vi "TestHarnessDPL-DetBoardOnly-MPCR-MP045-03.vi"() -> ()   [LabVIEW 2024]
uses:
  <vilib>/Analysis/6fits.llb/Curve Fitting Criteria.ctl
  <vilib>/Analysis/1siggen.llb/Ramp Pattern by Samples.vi
  <vilib>/Analysis/1siggen.llb/Ramp Pattern by Delta.vi
  <vilib>/Analysis/NI_AALBase.lvlib
  <userlib>/_OpenG.lib/time/time.llb/openg_time.lvlib
  <instrlib>/Detector SCPI/Detector SCPI.lvlib
  <instrlib>/Keithley 24XX/Keithley 24XX.lvlib
  <instrlib>/Keithley 648X Series/Keithley 648X Series.lvlib
  <vilib>/Analysis/NI_AALPro.lvlib
panel:
  out "error out":errorcluster
  out "OpVsCurrent":cluster{"Ramp Pattern":dbl[], dbl[]}[](array[cluster])
  in  "Abort 2":bool
  in  "Exit":bool
  in  "Measurement Mode":T1(tab)
  in  "DetectorData":T2(array[cluster])=[{"Name"="SWIR", "DAC Offset"=1800, "DAC StepsPerHGCount"=26.7}, {"Name"="MWIR", "DAC Offset"=666, "DAC StepsPerHGCount"=4.6}] {"DAC Offset" min=1 max=4095 step=1}
  in  "SPI Clock":i64=1000000
  in  "Oversample":i32=1 min=1 max=4096
  in  "Power":bool=TRUE
  in  "Detector VISA":refnum<visa-resource-name>="Detector_EGSE"
  out "Detector Resource":refnum<visa-resource-name>="COM4"
  out "Voltage (V)":dbl[](array[numeric])=[3.264, 0.0, 12.488, 12.77]
  out "Current (mA)":dbl[](array[numeric])=[0.0, 0.0, 21.6, -3.65]
  in  "ThrowAway":i32=100 min=1 max=10000
  out "Detector EGSE ID String":string="Aberystwyth University,Enfys Detector,#01,v0.5.0\r\n"
  in  "Current source":refnum<visa-resource-name>
  out "BoardTemperature":dbl
  in  "Tab Control":enum32{"Counts", "Temperature"}(tab)
  out "Counts":dbl(graph)=160.194
  out "Temperature":dbl(graph)=160.194
  in  "ResetVDACstats":bool
  in  "Gain":u16(ring) items=["High", "Med", "Low"]
  in  "DAC Value":i32=2076 min=0 max=4095 step=1
  in  "Detector":u16(ring) items=["SWIR", "MWIR"]
  out "Peak-to-Peak (counts)":dbl=0.0026870000001508743 format="%^.4g"
  out "rms (counts) 2":dbl=-2.7284841053187847e-12 format="%^.4g"
  out "Mean Value (counts)":dbl
  out "Elapsed(uS)":i32
  out "size":i32
  in  "Pause":bool
  out "XY Graph":cluster{dbl[], "subarray":dbl[]}(graph)
  in  "Detector 3":u16(ring) items=["SWIR", "MWIR"]
  in  "Gain 3":u16(ring) items=["High", "Med", "Low"]
  in  "trig":dbl=8.0 min=0.0 max=50.0
  in  "DetectorDAC":i32=2076 min=0 max=4095 step=1
  in  "Abort":bool
  out "Output vs current":cluster{"Ramp Pattern":dbl[], dbl[]}[](graph)
  in  "ISweep":bool
  in  "NPoints":i32=10 min=10 max=10000 step=1
  in  "MaxCurrent":dbl=1e-11 min=1e-11 max=1e-06
  in  "MinCurrent":dbl=1e-12 min=-10.0 max=10.0
  in  "Detector 4":u16(ring) items=["SWIR", "MWIR"]
  in  "LogSweep":bool
  in  "Gain 4":u16(ring) items=["High", "Med", "Low"]
  out "slope (counts/nA)":dbl
  out "intercept":dbl
  out "residue":dbl
  out "Max Deviation (counts)":dbl
  in  "DAC":i32 min=0 max=4095 step=1
  in  "Modulation Steps":i32=2 min=2 max=1000 step=1
  in  "Modulation Max":dbl min=0.0 max=10.0
  in  "Modulation Min":dbl min=-10.0 max=10.0
  in  "SweepLight":bool
  in  "Detector 7":u16(ring) items=["SWIR", "MWIR"]
  out "Output vs Light":cluster{dbl[], dbl[]}[](graph)
  in  "Gain 2":u16(ring) items=["High", "Med", "Low"]
  in  "SweepVDAC":bool
  in  "ISource":dbl min=-1e-06 max=1e-06
  in  "VDAC Step":i32=1 min=1 max=100
  in  "VDAC Max":i32 min=0 max=4095
  in  "VDAC Min":i32 min=0 max=4000
  in  "Detector 5":u16(ring) items=["SWIR", "MWIR"]
  out "VDAC Sweep":cluster{dbl[], dbl[]}[](graph)
  in  "Abort SweepVDAC":bool
  in  "Step":bool
  in  "Delay 1 (ms)":i32
  in  "Current 2":dbl
  in  "Current 1":dbl
  out "Step Response":cluster{dbl[], "subarray":dbl[]}(graph)
  in  "chan (0)":i32
  out "exit":bool=TRUE
  # "3.3V supply"
  # "Heater"
  # "+12V Supply"
  # "-12V Supply"
  # "Pause button will halt collection and display.\nThis allows graph to be printed etc."
  # "Burst mode is intended to examine behaviour of the ADC\n\nA burst of readings is recorded on the EGSE and then gathered here."
  # "Light source modulated by USB205L working as voltage source connected to MOD input of LD250C\nreference photodiode monitored by 6846 picoammeter"
  # "Set current to Current#1. Waits for Delay 1 to stabilise, then switches to current 2 and reads 1000 readings as fast as possible"
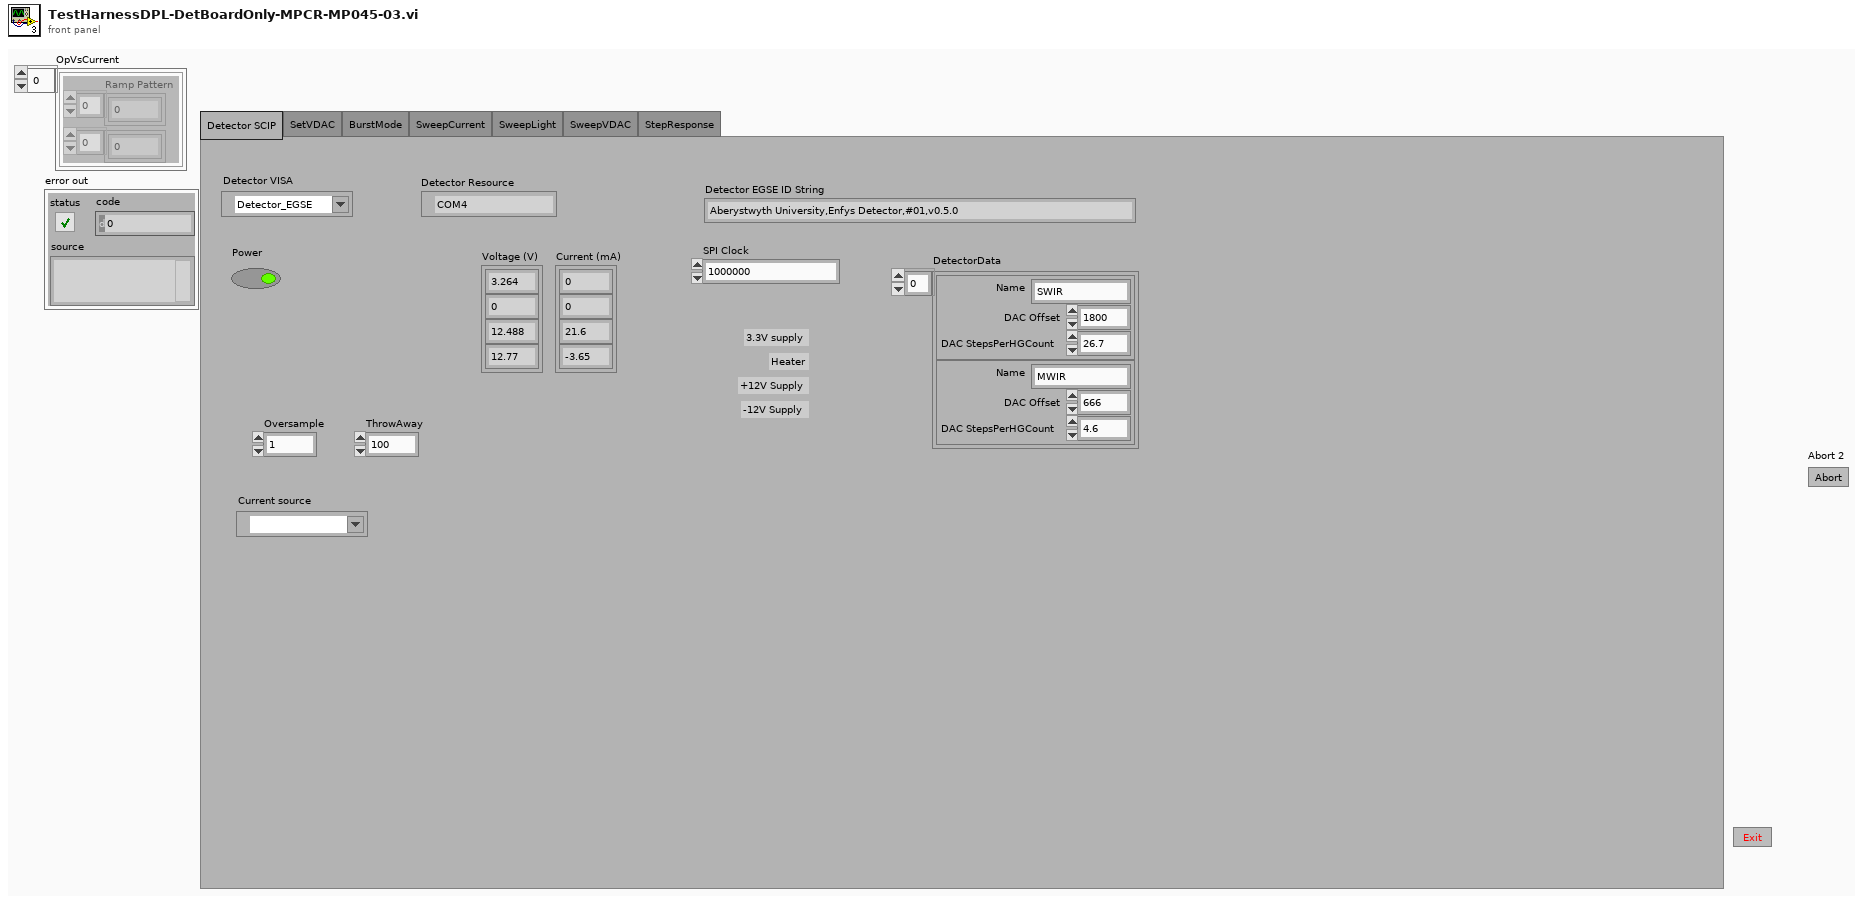
[diagram p1: front panel]
types:
  T1 = enum32{"Detector SCIP", "SetVDAC", "BurstMode", "SweepCurrent", "SweepLight", "SweepVDAC", "StepResponse"}
  T2 = cluster{"Name":string, "DAC Offset":i32, "DAC StepsPerHGCount":dbl}[]
  T3 = cluster{"Baud Rate":u32, "Parity":u16, "Data Bits":u16, "Stop Bits":u16, "Flow Control":u16}
  T4 = cluster{"Name":string, "DAC Offset":i32, "DAC StepsPerHGCount":dbl}
  T5 = typedef "NI_AALPro.lvlib/Curve Fitting Criteria.ctl" = u16
  T6 = typedef "LVPointDoubleTypeDef.ctl" = cluster{"Cursor X":dbl, "Cursor Y":dbl}
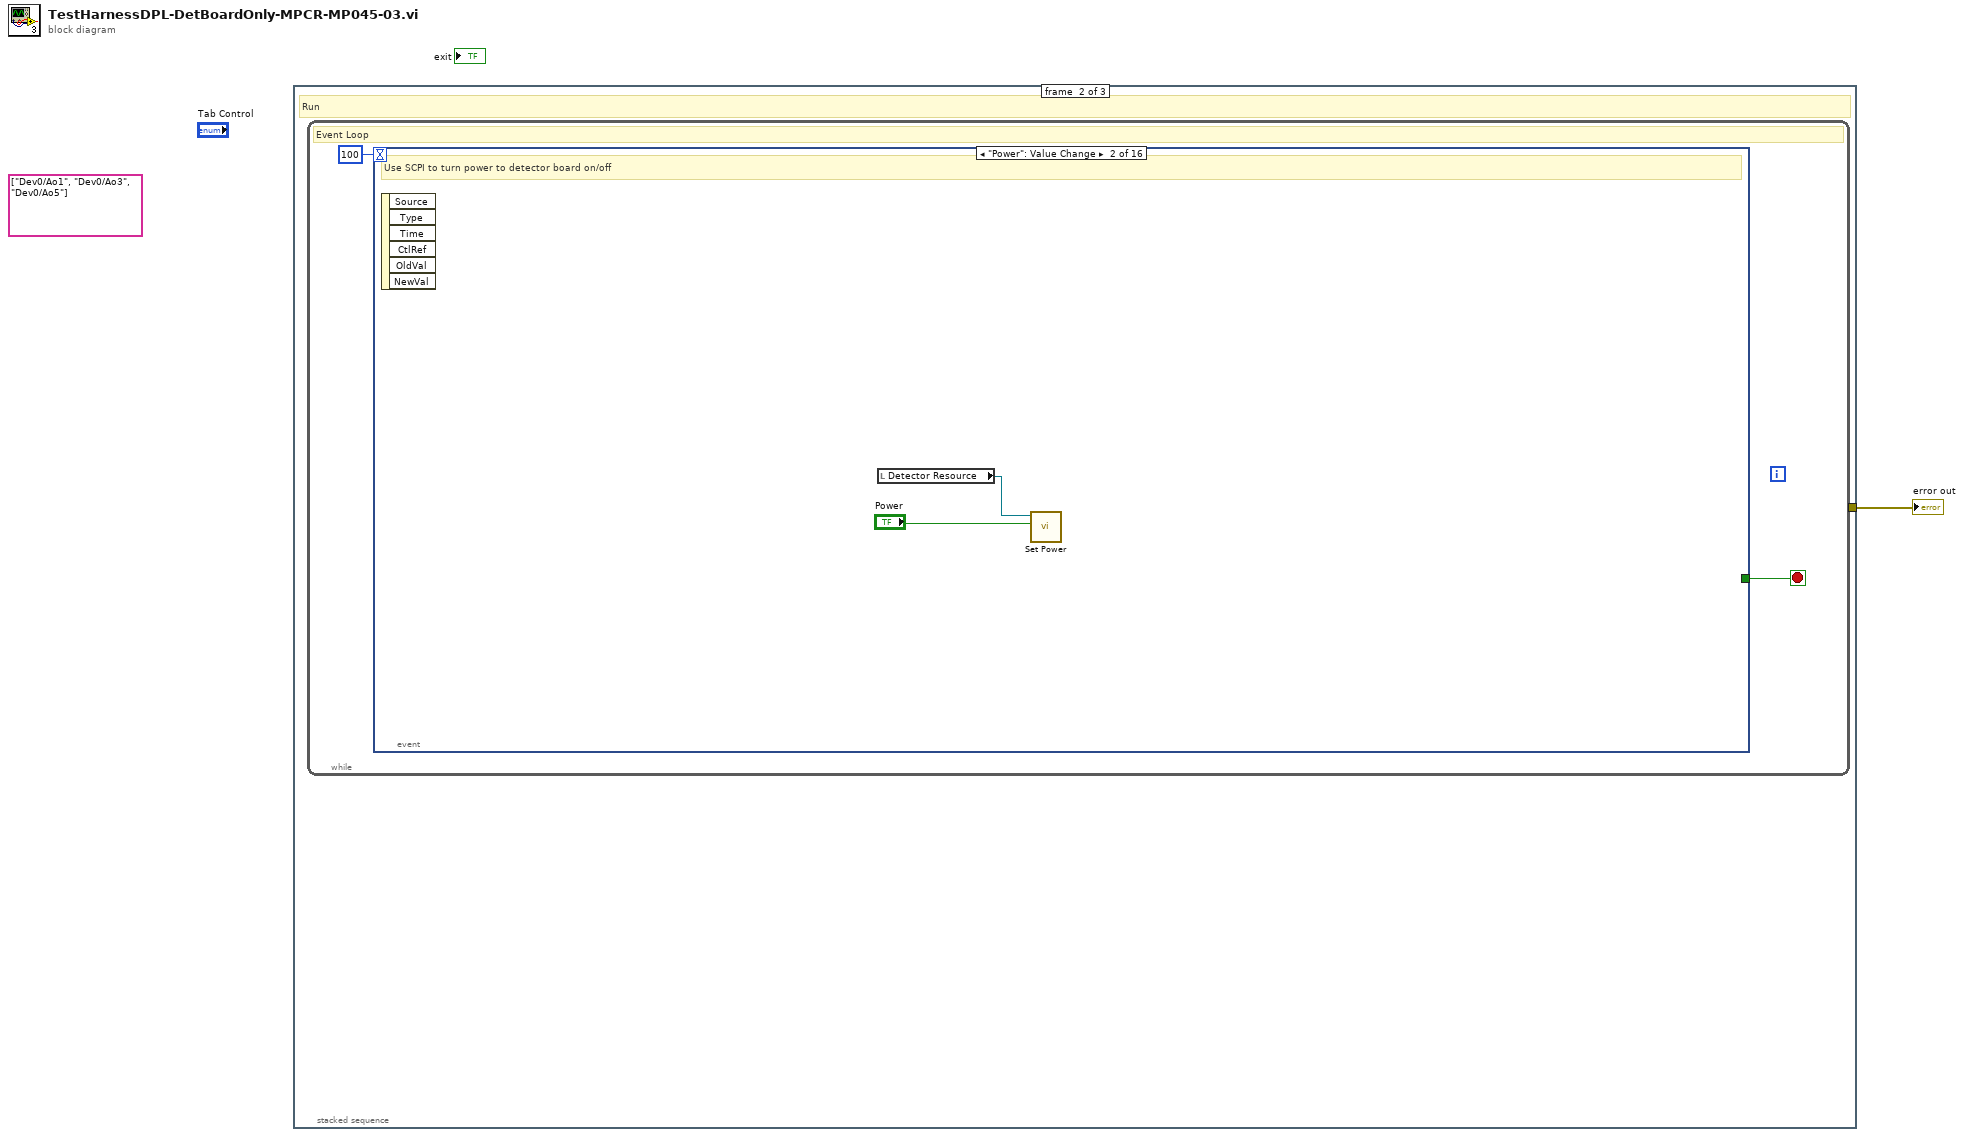
[diagram p0: block diagram]
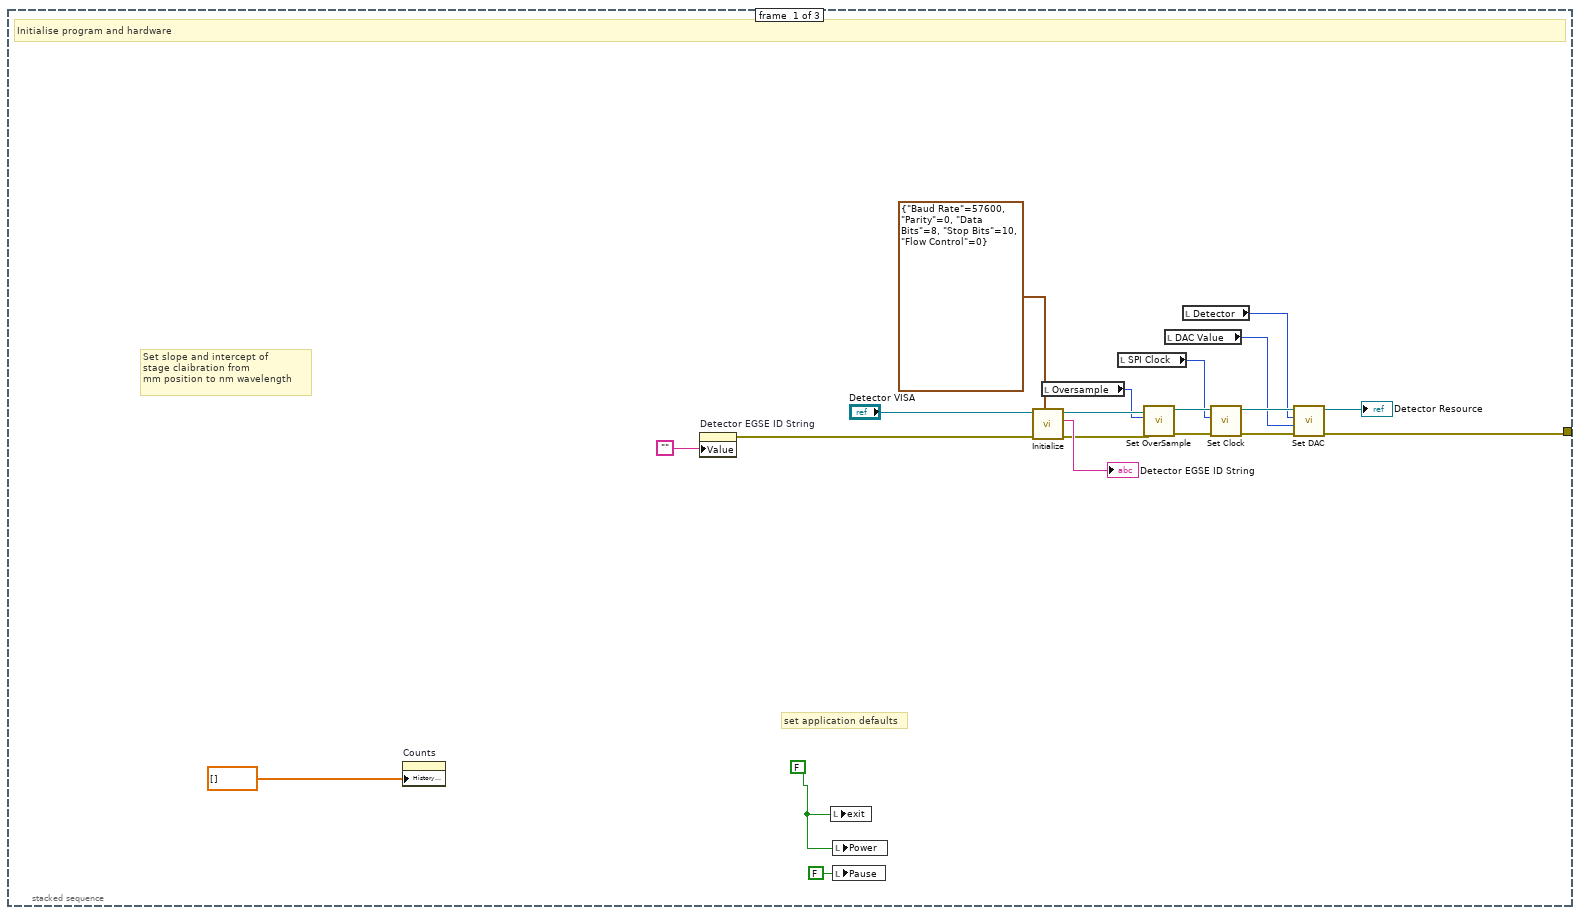
[diagram p2: hidden frame]
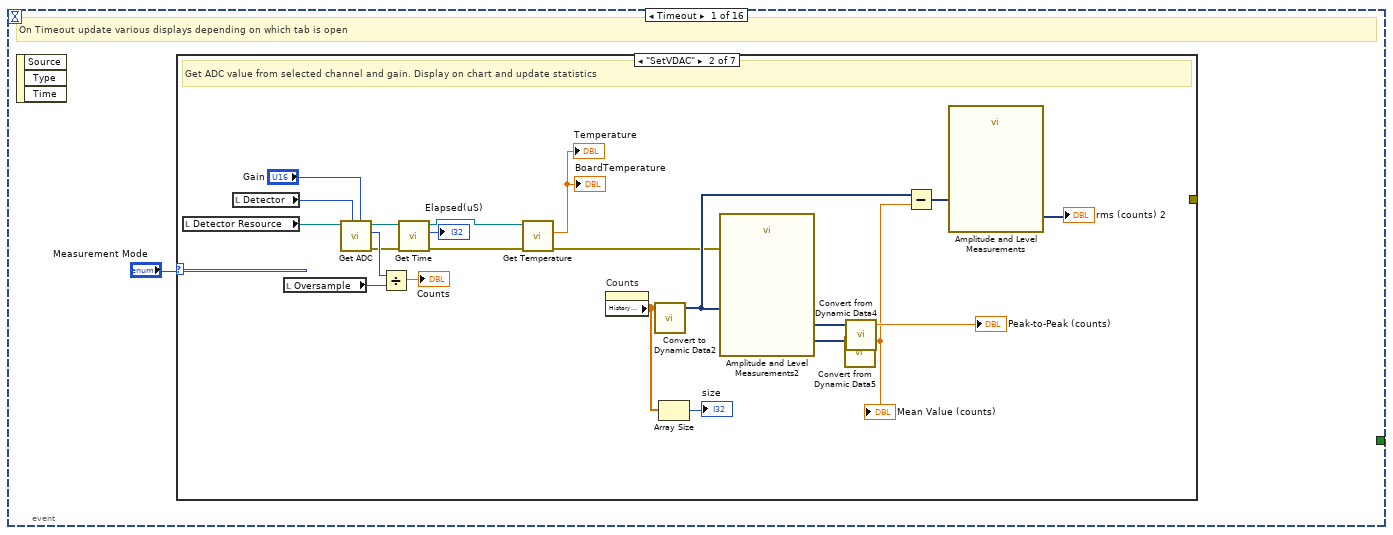
[diagram p3: hidden frame]
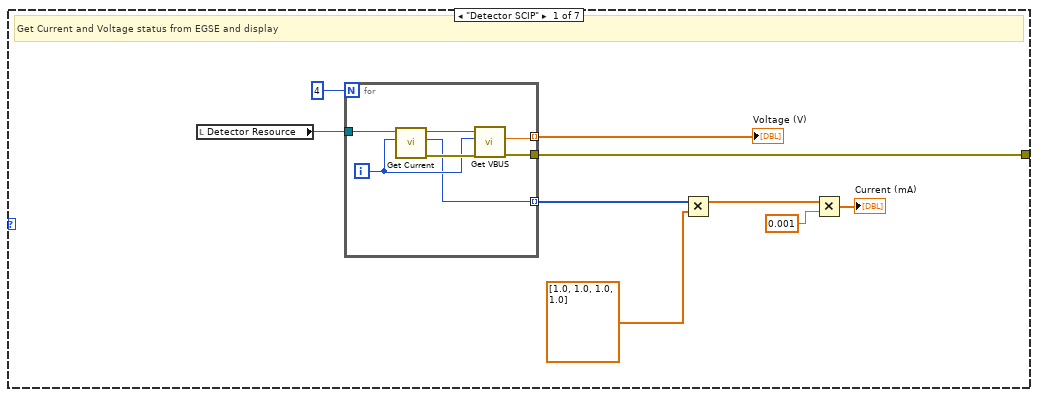
[diagram p4: hidden frame]
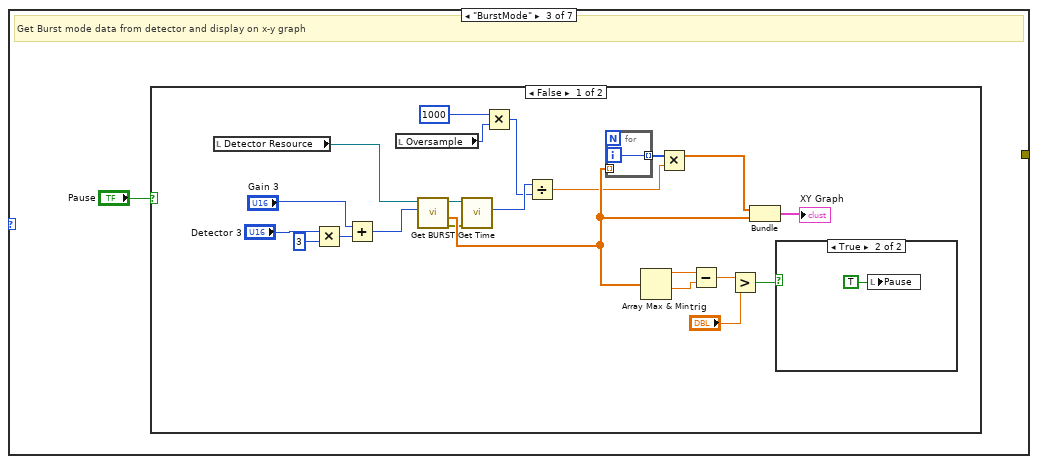
[diagram p5: hidden frame]
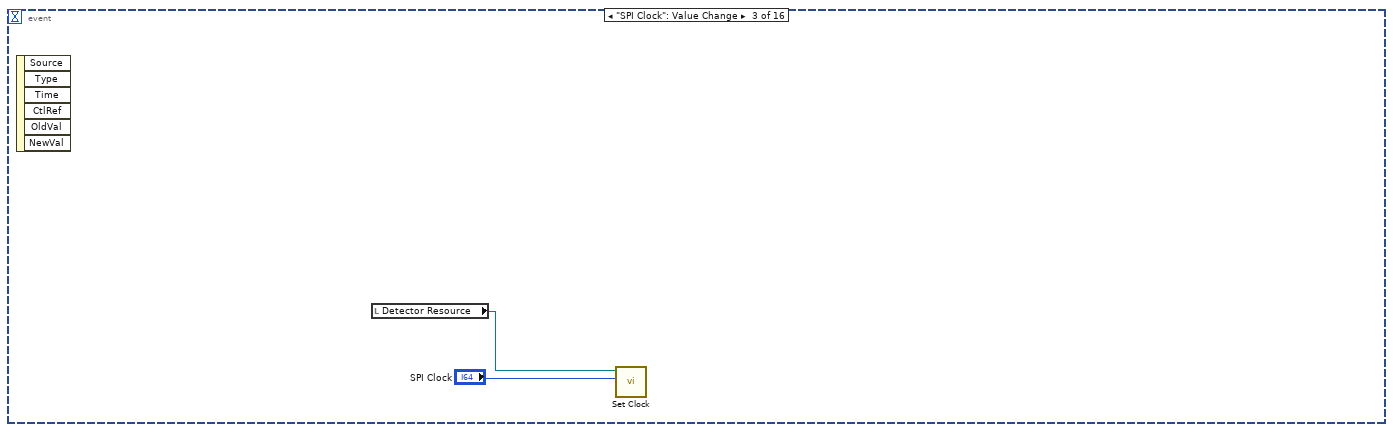
[diagram p12: hidden frame]
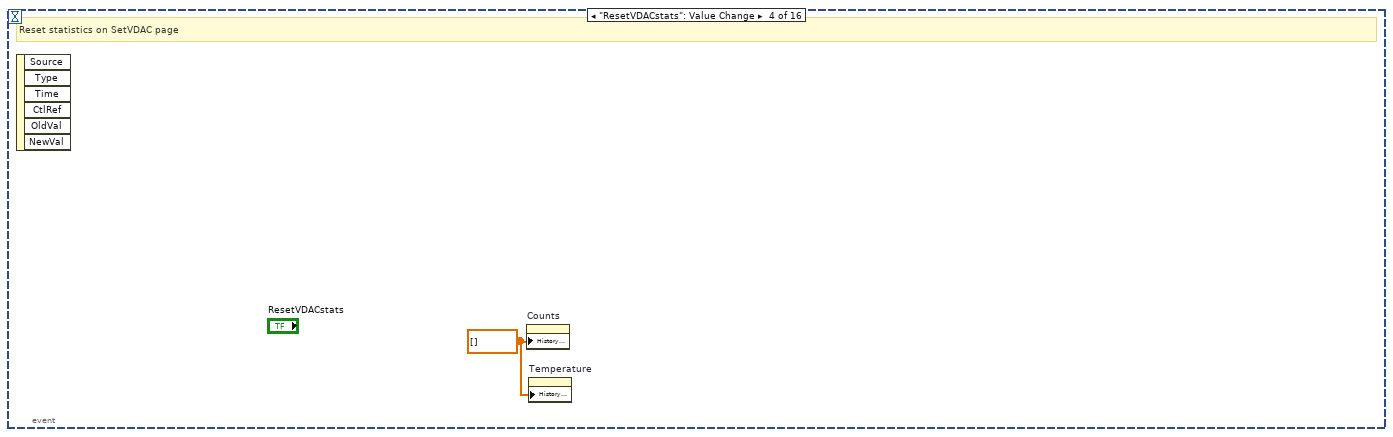
[diagram p13: hidden frame]
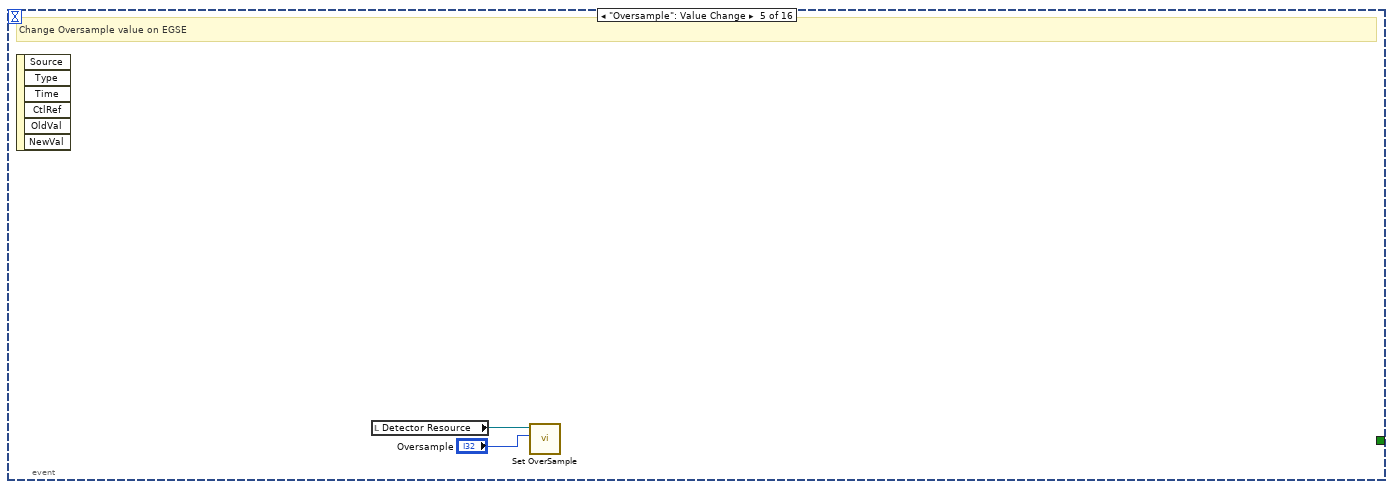
[diagram p14: hidden frame]
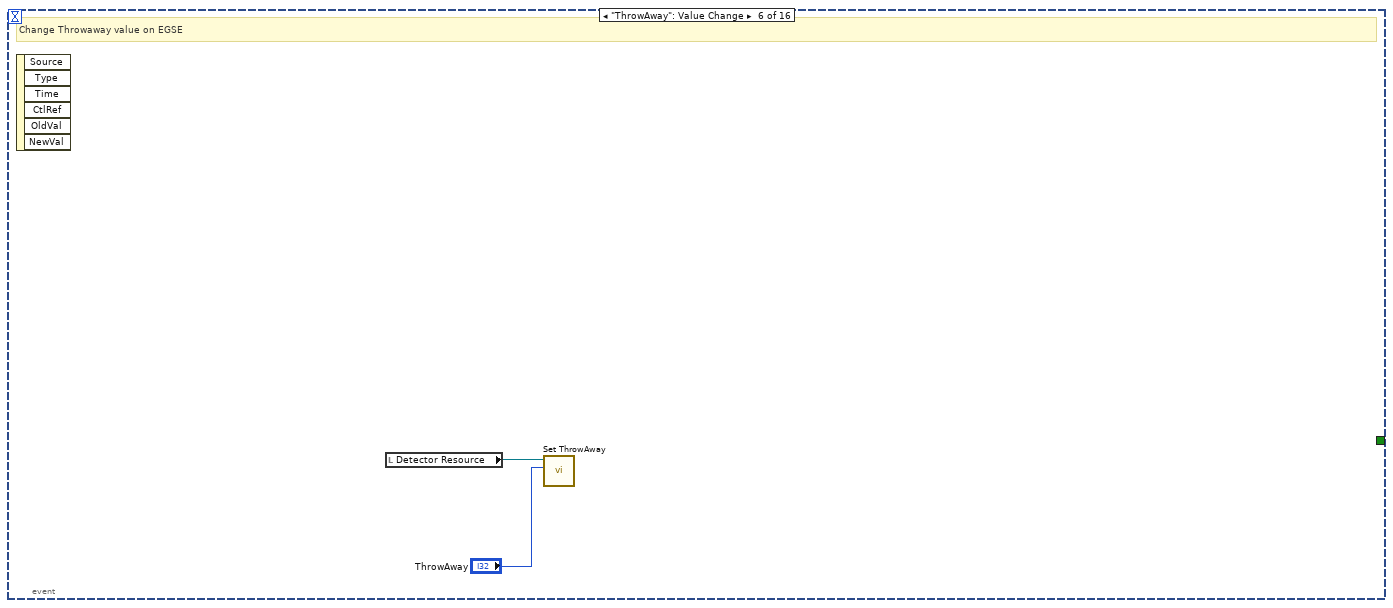
[diagram p15: hidden frame]
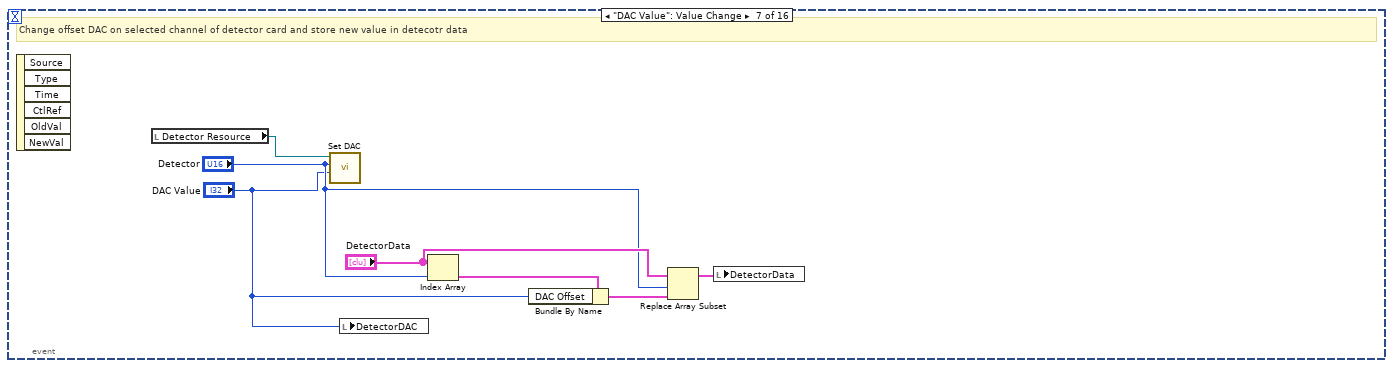
[diagram p16: hidden frame]
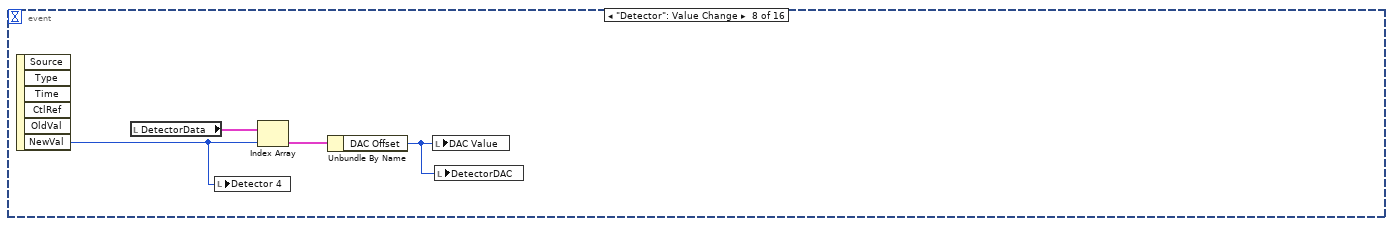
[diagram p17: hidden frame]
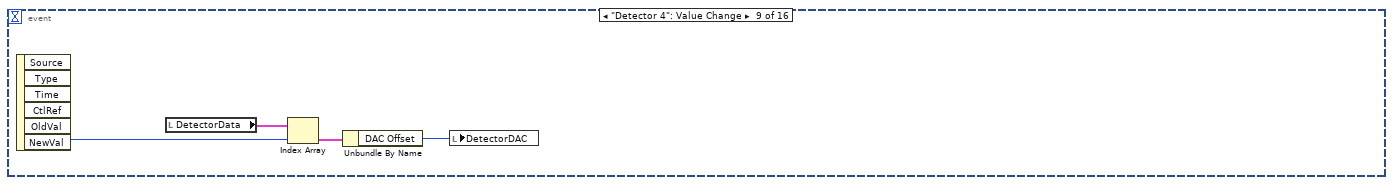
[diagram p18: hidden frame]
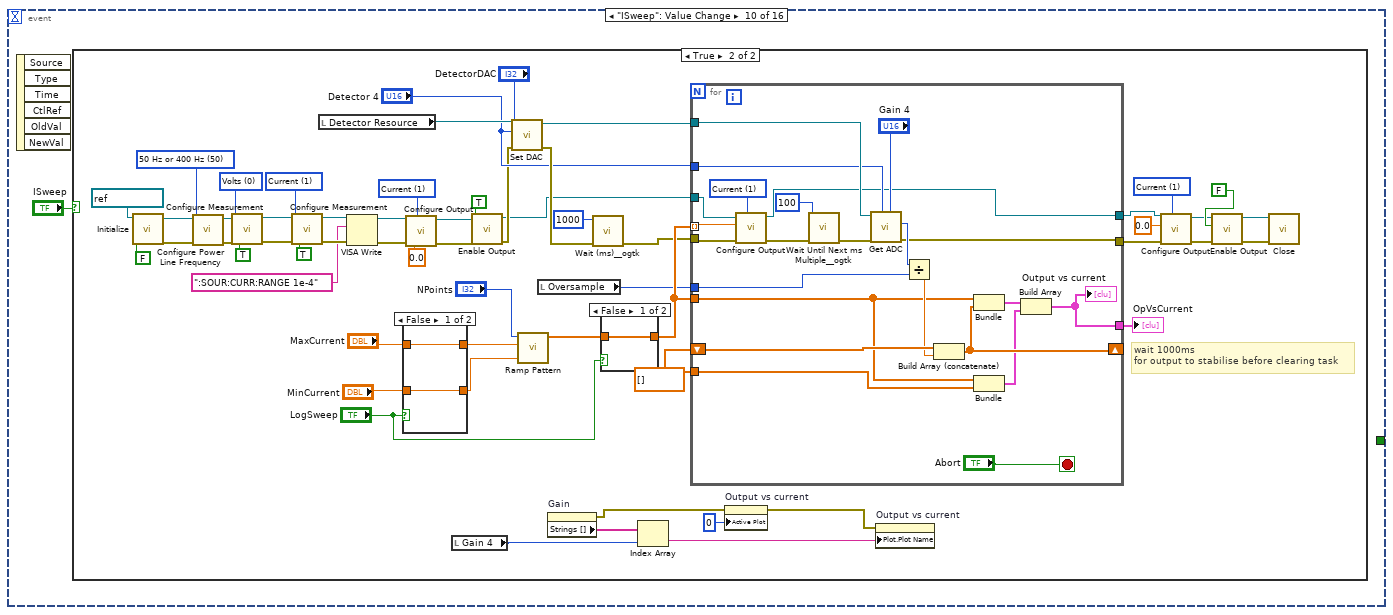
[diagram p19: hidden frame]
diagram:
  (unwired) string[] ["Dev0/Ao1", "Dev0/Ao3", "Dev0/Ao5"]
  n1 = stacked-sequence {
    tunnel: [w2 _ _] -> w1
    frame #0 {
      w20 = FALSE ("connected")
      # "Set slope and intercept of \nstage claibration from\nmm position to nm wavelength"
      # "set application defaults"
      # "Initialise program and hardware"
      n2 = property on="Counts" class="WFChart (strict)"("History Data"=dbl[] []) -> ()  [unwired: 2 in, 2 out]
      n3 = property on="Detector EGSE ID String" class="Str"("Value"="") -> (error out=w18:errorcluster)  [unwired: 2 in, 1 out]
      n4 = local write "exit"(w20) -> ()
      n5 = local write "Power"(w20) -> ()
      n6 = local write "Pause"(FALSE ("Pause")) -> ()
      n7 = call <instrlib>:"Initialize.vi"("Serial Configuration"=T3 {"Baud Rate"=57600, "Parity"=0, "Data Bits"=8, "Stop Bits"=10, "Flow Control"=0}, "error in (no error)"=w18, "VISA resource name"="Detector VISA") -> ("error out"=w14:errorcluster, "ID String"=→"Detector EGSE ID String":string, "VISA resource name out"=w13:refnum<visa-resource-name>)  [unwired: 6 in]
      n8 = local read "Oversample"() -> (w12:i32)
      n9 = local read "SPI Clock"() -> (w7:i64)
      n10 = call <instrlib>:"Set OverSample.vi"("error in (no error)"=w14, "oversample (0)"=w12, "VISA resource name"=w13) -> ("error out"=w11:errorcluster, "VISA resource name out"=w9:refnum<visa-resource-name>)  [unwired: 7 in]
      n11 = local read "DAC Value"() -> (w5:i32)
      n12 = local read "Detector"() -> (w6:u16)
      n13 = call <instrlib>:"Set Clock.vi"("error in (no error)"=w11, "ClockSpeed"=w7, "VISA resource name"=w9) -> ("error out"=w10:errorcluster, "VISA resource name out"=w8:refnum<visa-resource-name>)  [unwired: 7 in]
      n14 = call <instrlib>:"Set DAC.vi"("error in (no error)"=w10, "value (0)"=w5, "chan (0)"=w6, "VISA resource name"=w8) -> ("error out"=w2:errorcluster, "VISA resource name out"=→"Detector Resource":refnum<visa-resource-name>)  [unwired: 6 in]
    }
    frame #1 {
      # "Run"
      n15 = while {
        stop <- w22 stop-if-true
        # "Event Loop"
        n16 = event shown="[1] \"Power\": Value Change" {
          selector: _ -> [_ _ _ _ _ _ _ _ _ _ _ _ _ _ _ _]
          dyn-events: _ -> [_ _ _ _ _ _ _ _ _ _ _ _ _ _ _ _]
          timeout: 100 -> [_ _ _ _ _ _ _ _ _ _ _ _ _ _ _ _]
          tunnel: [_ _ _ _ _ _ _ _ _ _ _ _ _ _ "Exit" _] -> w22
          event Timeout {
            # "On Timeout update various displays depending on which tab is open"
            n17 = event-data() -> ()  [unwired: 1 in, 3 out]
            n18 = case shown="\"SetVDAC\"" "Measurement Mode" {
              tunnel: [w25 _ _ _ _ _ _] -> _
              frame "Detector SCIP" {
                # "Get Current and Voltage status from EGSE and display"
                n19 = local read "Detector Resource"() -> (w33:refnum<visa-resource-name>)
                n20 = for {
                  N: 4 -> [_]
                  tunnel: w33 -> [w40]
                  tunnel: [w36] -> w30 mode=indexing
                  tunnel: [w35] -> w31 mode=indexing
                  tunnel: [w34] -> w25
                  i -> [w37]
                  n21 = call <instrlib>:"Get Current.vi"("chan (1)"=w37, "VISA resource name"=w40) -> ("error out"=w39:errorcluster, "output"=w36:i32, "VISA resource name out"=w38:refnum<visa-resource-name>)  [unwired: 7 in]
                  n22 = call <instrlib>:"Get VBUS.vi"("error in (no error)"=w39, "chan (1)"=w37, "VISA resource name"=w38) -> ("error out"=w34:errorcluster, "output"=w35:dbl)  [unwired: 6 in, 1 out]
                }
                "Voltage (V)" <- w31
                n23 = Multiply(x=w30, y=dbl[] [1.0, 1.0, 1.0, 1.0]) -> (x*y=w27:dbl[])
                n24 = Multiply(x=w27, y=0.001) -> (x*y=→"Current (mA)":dbl[])
              }
              frame "SetVDAC" {
                # "Get ADC value from selected channel and gain. Display on chart and update statistics"
                n25 = local read "Detector Resource"() -> (w62:refnum<visa-resource-name>)
                n26 = local read "Detector"() -> (w57:u16)
                n27 = local read "Oversample"() -> (w59:i32)
                n28 = call <instrlib>:"Get ADC.vi"("Gain"="Gain", "Detector"=w57, "VISA resource name"=w62) -> ("error out"=w55:errorcluster, "output"=w61:i32, "VISA resource name out"=w56:refnum<visa-resource-name>)  [unwired: 6 in]
                n29 = Divide(x=w61, y=w59) -> (x/y=→"Counts":dbl)
                n30 = call <instrlib>:"Get Time.vi"("error in (no error)"=w55, "VISA resource name"=w56) -> ("error out"=w43:errorcluster, "output"=→"Elapsed(uS)":i32, "VISA resource name out"=w41:refnum<visa-resource-name>)  [unwired: 7 in]
                n31 = call <instrlib>:"Get Temperature.vi"("error in (no error)"=w43, "VISA resource name"=w41) -> ("error out"=w42:errorcluster, "output"=→"Temperature" →"BoardTemperature":dbl)  [unwired: 7 in, 1 out]
                n32 = property on="Counts" class="WFChart (strict)"() -> ("History Data"=w46:dbl[])  [unwired: 2 in, 2 out]
                n33 = call "Convert to Dynamic Data2"("Array"=w46) -> ("Dynamic Data Type"=w47:dynamicdata)  [unwired: 3 in]
                n34 = Array Size(array=w46) -> (size(s)=→"size":i32)
                n35 = call "Amplitude and Level Measurements2"("Signals"=w47, "error in (no error)"=w42) -> ("Mean (DC)"=w49:dynamicdata, "Peak to Peak"=w52:dynamicdata)  [unwired: 10 in, 2 out]
                n36 = call "Convert from Dynamic Data5"("Dynamic Data Type"=w49) -> ("Scalar"=w48:dbl)  [unwired: 3 in]
                "Mean Value (counts)" <- w48
                n37 = call "Convert from Dynamic Data4"("Dynamic Data Type"=w52) -> ("Scalar"=→"Peak-to-Peak (counts)":dbl)  [unwired: 3 in]
                n38 = Subtract(x=w47, y=w48) -> (x-y=w50:dynamicdata)
                n39 = call "Amplitude and Level Measurements"("Signals"=w50) -> ("RMS"=→"rms (counts) 2":dynamicdata)  [unwired: 11 in, 3 out]
              }
              frame "BurstMode" {
                # "Get Burst mode data from detector and display on x-y graph"
                n40 = case shown="False" "Pause" {
                  frame False {
                    n41 = local read "Detector Resource"() -> (w85:refnum<visa-resource-name>)
                    n42 = Multiply(x="Detector 3", y=u16 3) -> (x*y=w84:u16)
                    n43 = Add(x="Gain 3", y=w84) -> (x+y=w82:u16)
                    n44 = local read "Oversample"() -> (w69:i32)
                    n45 = call <instrlib>:"Get BURST.vi"("chan (0)"=w82, "VISA resource name"=w85) -> ("error out"=w71:errorcluster, "subarray"=w77:dbl[], "VISA resource name out"=w70:refnum<visa-resource-name>)  [unwired: 6 in, 1 out]
                    n46 = call <instrlib>:"Get Time.vi"("error in (no error)"=w71, "VISA resource name"=w70) -> ("output"=w68:i32)  [unwired: 7 in, 2 out]
                    n47 = Multiply(x=1000, y=w69) -> (x*y=w65:i32)
                    n48 = Divide(x=w68, y=w65) -> (x/y=w66:dbl)
                    n49 = for {
                      tunnel: w77 -> [_] mode=indexing
                      tunnel: [w87] -> w78 mode=indexing
                      i -> [w87]
                    }
                    n50 = Array Max & Min(array=w77) -> (max value=w76:dbl, min value=w75:dbl)  [unwired: 2 out]
                    n51 = Multiply(x=w78, y=w66) -> (x*y=w67:dbl[])
                    n52 = Subtract(x=w76, y=w75) -> (x-y=w74:dbl)
                    n53 = Greater?(x=w74, y="trig") -> (0:w72:bool)
                    n54 = Bundle(w67, "subarray"=w77) -> (→"XY Graph":cluster{dbl[], "subarray":dbl[]})  [unwired: 1 in]
                    n55 = case shown="True" w72 {
                      frame False {
                      }
                      frame True {
                        n56 = local write "Pause"(TRUE ("Pause")) -> ()
                      }
                    }
                  }
                  frame True {
                  }
                }
              }
              frame "SweepCurrent" {
              }
              frame "SweepVDAC" {
              }
              frame "StepResponse" {
              }
              frame "SweepLight" {
              }
            }
          }
          event "Power": Value Change {
            # "Use SCPI to turn power to detector board on/off"
            n57 = event-data() -> ()  [unwired: 1 in, 6 out]
            n58 = local read "Detector Resource"() -> (w89:refnum<visa-resource-name>)
            n59 = call <instrlib>:"Set Power.vi"("Power (0)"="Power", "VISA resource name"=w89) -> ()  [unwired: 8 in, 2 out]
          }
          event "SPI Clock": Value Change {
            n60 = event-data() -> ()  [unwired: 1 in, 6 out]
            n61 = local read "Detector Resource"() -> (w91:refnum<visa-resource-name>)
            n62 = call <instrlib>:"Set Clock.vi"("ClockSpeed"="SPI Clock", "VISA resource name"=w91) -> ()  [unwired: 8 in, 2 out]
          }
          event "ResetVDACstats": Value Change {
            w92 = dbl[] [] ("History Data")
            # "Reset statistics on SetVDAC page"
            n63 = event-data() -> ()  [unwired: 1 in, 6 out]
            n64 = property on="Counts" class="WFChart (strict)"("History Data"=w92) -> ()  [unwired: 2 in, 2 out]
            n65 = property on="Temperature" class="WFChart (strict)"("History Data"=w92) -> ()  [unwired: 2 in, 2 out]
          }
          event "Oversample": Value Change {
            # "Change Oversample value on EGSE"
            n66 = event-data() -> ()  [unwired: 1 in, 6 out]
            n67 = local read "Detector Resource"() -> (w94:refnum<visa-resource-name>)
            n68 = call <instrlib>:"Set OverSample.vi"("oversample (0)"="Oversample", "VISA resource name"=w94) -> ()  [unwired: 8 in, 2 out]
          }
          event "ThrowAway": Value Change {
            # "Change Throwaway value on EGSE"
            n69 = event-data() -> ()  [unwired: 1 in, 6 out]
            n70 = local read "Detector Resource"() -> (w96:refnum<visa-resource-name>)
            n71 = call <instrlib>:"Set ThrowAway.vi"("ThrowAway (0)"="ThrowAway", "VISA resource name"=w96) -> ()  [unwired: 8 in, 2 out]
          }
          event "DAC Value": Value Change {
            # "Change offset DAC on selected channel of detector card and store new value in detecotr data"
            n72 = event-data() -> ()  [unwired: 1 in, 6 out]
            n73 = local read "Detector Resource"() -> (w103:refnum<visa-resource-name>)
            n74 = call <instrlib>:"Set DAC.vi"("value (0)"="DAC Value", "chan (0)"="Detector", "VISA resource name"=w103) -> ()  [unwired: 7 in, 2 out]
            n75 = local write "DetectorDAC"("DAC Value") -> ()
            n76 = Index Array(array="DetectorData", index="Detector") -> (element=w102:T4)
            n77 = Bundle By Name(cluster=w102, "DAC Offset"="DAC Value") -> (w99:T4)
            n78 = Replace Array Subset(array="DetectorData", new element=w99, index="Detector") -> (w98:T2)
            n79 = local write "DetectorData"(w98) -> ()
          }
          event "Detector": Value Change {
            n80 = event-data() -> ("NewVal"=w104:u16)  [unwired: 1 in, 5 out]
            n81 = local read "DetectorData"() -> (w107:T2)
            n82 = local write "Detector 4"(w104) -> ()
            n83 = Index Array(array=w107, index=w104) -> (element=w106:T4)
            n84 = Unbundle By Name(w106) -> ("DAC Offset"=w105:i32)
            n85 = local write "DAC Value"(w105) -> ()
            n86 = local write "DetectorDAC"(w105) -> ()
          }
          event "Detector 4": Value Change {
            n87 = event-data() -> ("NewVal"=w110:u16)  [unwired: 1 in, 5 out]
            n88 = local read "DetectorData"() -> (w111:T2)
            n89 = Index Array(array=w111, index=w110) -> (element=w109:T4)
            n90 = Unbundle By Name(w109) -> ("DAC Offset"=w108:i32)
            n91 = local write "DetectorDAC"(w108) -> ()
          }
          event "ISweep": Value Change {
            n92 = event-data() -> ()  [unwired: 1 in, 6 out]
            n93 = case shown="True" "ISweep" {
              frame False {
              }
              frame True {
                w118 = u16 50 items=["60 Hz"=60, "50 Hz or 400 Hz"=50] ("Power Line Frequency  (60 Hz)")
                w128 = u16 1 items=["Voltage", "Current"] ("Source Mode  (0: Voltage)")
                w137 = u16 1 items=["Volts", "Current", "Resistance"] ("Function (0: Volts)")
                w140 = u16 0 items=["Volts", "Current", "Resistance"] ("Function (0: Volts)")
                w144 = u16 1 items=["Voltage", "Current"] ("Source Mode  (0: Voltage)")
                w155 = dbl[] []
                # "wait 1000ms\nfor output to stabilise before clearing task"
                n94 = call <instrlib>:"Initialize.vi"("ID Query (True)"=FALSE, "VISA resource name"=refnum<visa-resource-name> "B2901BL") -> ("error out"=w119:errorcluster, "VISA resource name out"=w122:refnum<visa-resource-name>)  [unwired: 8 in]
                n95 = call <instrlib>:"Configure Power Line Frequency.vi"("error in (no error)"=w119, "Power Line Frequency  (60 Hz)"=w118, "VISA resource name"=w122) -> ("error out"=w120:errorcluster, "VISA resource name out"=w121:refnum<visa-resource-name>)  [unwired: 7 in]
                n96 = call <instrlib>:"Configure Measurement.vi"("error in (no error)"=w120, "Enable Auto Range (T:Enable)"=TRUE, "Function (0: Volts)"=w140, "VISA resource name"=w121) -> ("error out"=w135:errorcluster, "VISA resource name out"=w136:refnum<visa-resource-name>)  [unwired: 6 in]
                n97 = call <instrlib>:"Configure Measurement.vi"("error in (no error)"=w135, "Enable Auto Range (T:Enable)"=TRUE, "Function (0: Volts)"=w137, "VISA resource name"=w136) -> ("error out"=w117:errorcluster, "VISA resource name out"=w116:refnum<visa-resource-name>)  [unwired: 6 in]
                n98 = local read "Detector Resource"() -> (w162:refnum<visa-resource-name>)
                n99 = VISA Write(VISA resource name=w116, write buffer=":SOUR:CURR:RANGE 1e-4", error in (no error)=w117) -> (VISA resource name out=w115:refnum<visa-resource-name>, error out=w114:errorcluster)  [unwired: 1 out]
                n100 = case shown="False" "LogSweep" {
                  tunnel: "MaxCurrent" -> [w172 w176]
                  tunnel: "MinCurrent" -> [w171 w175]
                  tunnel: [w172 w174] -> w166
                  tunnel: [w171 w173] -> w165
                  frame False {
                  }
                  frame True {
                    n101 = Logarithm Base 10(1:w176) -> (0:w174:dbl)
                    n102 = Logarithm Base 10(1:w175) -> (0:w173:dbl)
                  }
                }
                n103 = call <instrlib>:"Configure Output.vi"("Source Mode  (0: Voltage)"=w144, "error in (no error)"=w114, "Output Level (0)"=0.0, "VISA resource name"=w115) -> ("error out"=w143:errorcluster, "VISA resource name out"=w142:refnum<visa-resource-name>)  [unwired: 6 in]
                n104 = local read "Gain 4"() -> (w147:u16)
                n105 = call <instrlib>:"Enable Output.vi"("error in (no error)"=w143, "Enable Output (T: Enable)"=TRUE ("Auto Output-Off (F: Disable)"), "VISA resource name"=w142) -> ("error out"=w133:errorcluster, "VISA resource name out"=w132:refnum<visa-resource-name>)  [unwired: 7 in]
                n106 = call <instrlib>:"Set DAC.vi"("error in (no error)"=w133, "value (0)"="DetectorDAC", "chan (0)"="Detector 4", "VISA resource name"=w162) -> ("error out"=w157:errorcluster, "VISA resource name out"=w161:refnum<visa-resource-name>)  [unwired: 6 in]
                n107 = call-poly <vilib>:"Ramp Pattern.vi"("start"=w165, "end"=w166, "samples"="NPoints") -> ("Ramp Pattern"=w167:dbl[])  [unwired: 7 in, 1 out]
                n108 = local read "Oversample"() -> (w163:i32)
                n109 = property on="Gain" class="Ring (strict)"() -> (error out=w148:errorcluster, "Strings []"=w153:string[])  [unwired: 2 in, 1 out]
                n110 = call <userlib>:"Wait (ms)__ogtk.vi"("error in (no error)"=w157, "milliseconds to wait"=u32 1000) -> ("error out"=w158:errorcluster)  [unwired: 8 in, 1 out]
                n111 = case shown="False" "LogSweep" {
                  tunnel: w167 -> [w177 w179]
                  tunnel: [w177 w178] -> w164
                  frame False {
                  }
                  frame True {
                    n112 = Power Of 10(x=w179) -> (10^x=w178:dbl[])
                  }
                }
                n113 = Index Array(array=w153, index=w147) -> (element=w149:string)
                n114 = for {
                  tunnel: w158 -> [w193]
                  tunnel: w164 -> [w182] mode=indexing
                  tunnel: [w191] -> w123
                  shift-right: [w199] -> _
                  shift-left: w155 -> [w201]
                  tunnel: w164 -> [w186]
                  tunnel: w161 -> [w198]
                  tunnel: w163 -> [w195]
                  tunnel: "Detector 4" -> [w194]
                  tunnel: [w192] -> w124
                  tunnel: [w184] -> w154
                  tunnel: w155 -> [w185]
                  tunnel: w132 -> [w180]
                  stop <- "Abort" stop-if-true
                  w181 = u16 1 items=["Voltage", "Current"] ("Source Mode  (0: Voltage)")
                  n115 = call <instrlib>:"Configure Output.vi"("Source Mode  (0: Voltage)"=w181, "error in (no error)"=w193, "Output Level (0)"=w182, "VISA resource name"=w180) -> ("error out"=w190:errorcluster, "VISA resource name out"=w192:refnum<visa-resource-name>)  [unwired: 6 in]
                  n116 = call <userlib>:"Wait Until Next ms Multiple__ogtk.vi"("error in (no error)"=w190, "milliseconds to wait"=u32 100) -> ("error out"=w189:errorcluster)  [unwired: 8 in, 1 out]
                  n117 = call <instrlib>:"Get ADC.vi"("Gain"="Gain 4", "Detector"=w194, "error in (no error)"=w189, "VISA resource name"=w198) -> ("error out"=w191:errorcluster, "output"=w200:i32)  [unwired: 5 in, 1 out]
                  n118 = Divide(x=w200, y=w195) -> (x/y=w196:dbl)
                  n119 = Build Array (concatenate)(w201, w196) -> (w199:dbl[])
                  n120 = Bundle("Ramp Pattern"=w186, w199) -> (w187:cluster{"Ramp Pattern":dbl[], dbl[]})  [unwired: 1 in]
                  n121 = Bundle("Ramp Pattern"=w186, w185) -> (w183:cluster{"Ramp Pattern":dbl[], dbl[]})  [unwired: 1 in]
                  n122 = Build Array(w187, w183) -> (w184:cluster{"Ramp Pattern":dbl[], dbl[]}[])
                  "Output vs current" <- w184
                }
                "OpVsCurrent" <- w154
                n123 = property on="Output vs current" class="XYGraph (strict)"(error in=w148, "Active Plot"=u32 0) -> (error out=w150:errorcluster)  [unwired: 1 in, 1 out]
                n124 = property on="Output vs current" class="XYGraph (strict)"(error in=w150, "Plot.Plot Name"=w149) -> ()  [unwired: 1 in, 2 out]
                n125 = call <instrlib>:"Configure Output.vi"("Source Mode  (0: Voltage)"=w128, "error in (no error)"=w123, "Output Level (0)"=0.0, "VISA resource name"=w124) -> ("error out"=w126:errorcluster, "VISA resource name out"=w125:refnum<visa-resource-name>)  [unwired: 6 in]
                n126 = call <instrlib>:"Enable Output.vi"("error in (no error)"=w126, "Enable Output (T: Enable)"=FALSE ("Auto Output-Off (F: Disable)"), "VISA resource name"=w125) -> ("error out"=w130:errorcluster, "VISA resource name out"=w131:refnum<visa-resource-name>)  [unwired: 7 in]
                n127 = call <instrlib>:"Close.vi"("error in (no error)"=w130, "VISA resource name"=w131) -> ()  [unwired: 9 in, 1 out]
              }
            }
          }
          event "Output vs current": Cursor Release {
            w221 = T5 0 items=["Least Square", "Least Absolute Residual", "Bisquare"] ("method")
            n128 = event-data() -> ()  [unwired: 1 in, 9 out]
            n129 = property on="Output vs current" class="XYGraph (strict)"("Active Cursor"=u32 0) -> (error out=w233:errorcluster)  [unwired: 2 in, 1 out]
            n130 = property on="Output vs current" class="XYGraph (strict)"(error in=w233) -> (error out=w230:errorcluster, "Cursor.Cursor Position"=w228:T6)  [unwired: 1 in, 1 out]
            n131 = Unbundle By Name(w228) -> ("Cursor X"=w216:dbl)
            n132 = local read "OpVsCurrent"() -> (w229:cluster{"Ramp Pattern":dbl[], dbl[]}[])
            n133 = property on="Output vs current" class="XYGraph (strict)"(error in=w230, "Active Cursor"=u32 1) -> (error out=w232:errorcluster)  [unwired: 1 in, 1 out]
            n134 = Index Array(array=w229) -> (element=w213:cluster{"Ramp Pattern":dbl[], dbl[]})  [unwired: 1 in]
            n135 = property on="Output vs current" class="XYGraph (strict)"(error in=w232) -> ("Cursor.Cursor Position"=w227:T6)  [unwired: 1 in, 2 out]
            n136 = Unbundle(w213) -> ("Ramp Pattern"=w226:dbl[], w224:dbl[])
            n137 = Unbundle By Name(w227) -> ("Cursor X"=w217:dbl)
            n138 = Max & Min(x=w217, y=w216) -> (max(x,y)=w214:dbl, min(x,y)=w215:dbl)
            n139 = Search 1D Array(1D array=w226, element=w215) -> (index of element=w223:i32)  [unwired: 1 in]
            n140 = local read "Output vs current"() -> (w211:cluster{"Ramp Pattern":dbl[], dbl[]}[])
            n141 = Search 1D Array(1D array=w226, element=w214) -> (index of element=w225:i32)  [unwired: 1 in]
            n142 = Subtract(x=w225, y=w223) -> (x-y=w222:i32)
            n143 = Array Subset(array=w224, index=w223, length=w222) -> (w206:dbl[])
            n144 = Array Subset(array=w226, index=w223, length=w222) -> (w212:dbl[])
            n145 = call <vilib>:"Linear Fit.vi"("Y"=w206, "X"=w212, "method"=w221) -> ("Best Linear Fit"=w207:dbl[], "slope"=→"slope (counts/nA)":dbl, "intercept"=→"intercept":dbl, "residue"=→"residue":dbl)  [unwired: 8 in, 1 out]
            n146 = Bundle(w212, "Best Linear Fit"=w207) -> (w209:cluster{dbl[], "Best Linear Fit":dbl[]})  [unwired: 1 in]
            n147 = Replace Array Subset(array=w211, new element=w209, index=1) -> (w208:cluster{"Ramp Pattern":dbl[], dbl[]}[])
            n148 = Subtract(x=w206, y=w207) -> (x-y=w205:dbl[])
            n149 = local write "Output vs current"(w208) -> ()
            n150 = Absolute Value(x=w205) -> (abs(x)=w204:dbl[])
            n151 = Array Max & Min(array=w204) -> (max value=→"Max Deviation (counts)":dbl)  [unwired: 3 out]
          }
          event "SweepLight": Value Change {
            n152 = event-data() -> ()  [unwired: 1 in, 6 out]
            n153 = case shown="True" "SweepLight" {
              frame False {
              }
              frame True {
                w252 = dbl[] []
                n154 = local read "Detector Resource"() -> (w261:refnum<visa-resource-name>)
                n155 = call "Keithley 648X Series SetupAcquisition.vi"("VISA resource name"=refnum<visa-resource-name> "Picoammeter") -> ("VISA resource name out"=w253:refnum<visa-resource-name>)  [unwired: 8 in, 1 out]
                n156 = local read "Oversample"() -> (w262:i32)
                n157 = call-poly <vilib>:"Ramp Pattern.vi"("start"="Modulation Min", "end"="Modulation Max", "samples"="Modulation Steps") -> ("Ramp Pattern"=w257:dbl[])  [unwired: 7 in, 1 out]
                n158 = call <instrlib>:"Set DAC.vi"("value (0)"="DAC", "chan (0)"="Detector 7", "VISA resource name"=w261) -> ("error out"=w251:errorcluster, "VISA resource name out"=w260:refnum<visa-resource-name>)  [unwired: 7 in]
                n159 = call <instrlib>:"ULx Create Channel (AO-Voltage-Basic).vi"("maximum value"=5.0, "minimum value"=0.0, "physical channels"=refnum<k21> "Dev0/Ao0", "error in"=w251) -> ("task out"=w246:refnum<k24>, "error out"=w245:errorcluster)  [unwired: 10 in]
                n160 = call <instrlib>:"ULx Write (Analog 1D DBL 1Chan 1Samp).vi"("task in"=w246, "data"="Modulation Min", "error in"=w245) -> ("task out"=w247:refnum<k24>, "error out"=w242:errorcluster)  [unwired: 10 in, 1 out]
                n161 = call <userlib>:"Wait (ms)__ogtk.vi"("error in (no error)"=w242, "milliseconds to wait"=u32 1000) -> ("error out"=w243:errorcluster)  [unwired: 8 in, 1 out]
                n162 = for {
                  tunnel: w243 -> [w291]
                  tunnel: [w290] -> w237
                  tunnel: [w272] -> w239
                  shift-right: [w285] -> _
                  shift-left: w252 -> [w287]
                  tunnel: w260 -> [w284]
                  shift-right: [w280] -> _
                  shift-left: w252 -> [w282]
                  shift-right: [w279] -> _
                  shift-left: w252 -> [w281]
                  tunnel: w262 -> [w274]
                  tunnel: "Detector 7" -> [w273]
                  tunnel: w257 -> [w265] mode=indexing
                  tunnel: w253 -> [w271]
                  shift-right: [w267] -> _
                  shift-left: w252 -> [w268]
                  tunnel: w247 -> [w266]
                  stop <- "Abort 2" stop-if-true
                  n163 = call <instrlib>:"ULx Write (Analog 1D DBL 1Chan 1Samp).vi"("task in"=w266, "data"=w265, "error in"=w291) -> ("task out"=w290:refnum<k24>, "error out"=w289:errorcluster)  [unwired: 10 in, 1 out]
                  n164 = call <instrlib>:"Get ADC.vi"("Gain"="Gain 2", "Detector"=w273, "error in (no error)"=w289, "VISA resource name"=w284) -> ("error out"=w283:errorcluster, "output"=w286:i32)  [unwired: 5 in, 1 out]
                  n165 = Divide(x=w286, y=w274) -> (x/y=w263:dbl)
                  n166 = Divide(x=w273, y=w274) -> ()  [unwired: 1 out]
                  n167 = Build Array (concatenate)(w282, w263) -> (w280:dbl[])
                  n168 = Build Array (concatenate)(w287, w263) -> (w285:dbl[])
                  n169 = Build Array (concatenate)(w281, w263) -> (w279:dbl[])
                  n170 = call <instrlib>:"Measure Current.vi"("VISA resource name"=w271, "error in (no error)"=w283) -> ("Measurement"=w269:dbl, "error out"=w272:errorcluster)  [unwired: 11 in, 1 out]
                  n171 = Negate(x=w269) -> (-x=w264:dbl)
                  n172 = Build Array (concatenate)(w268, w264) -> (w267:dbl[])
                  n173 = Bundle(w267, w285) -> (w278:cluster{dbl[], dbl[]})  [unwired: 1 in]
                  n174 = Bundle(w267, w280) -> (w277:cluster{dbl[], dbl[]})  [unwired: 1 in]
                  n175 = Bundle(w267, w279) -> (w276:cluster{dbl[], dbl[]})  [unwired: 1 in]
                  n176 = Build Array(w278, w277, w276) -> (→"Output vs Light":cluster{dbl[], dbl[]}[])
                }
                n177 = call <instrlib>:"ULx Write (Analog 1D DBL 1Chan 1Samp).vi"("task in"=w237, "data"=0.0, "error in"=w239) -> ("task out"=w238:refnum<k24>, "error out"=w240:errorcluster)  [unwired: 10 in, 1 out]
                n178 = call <instrlib>:"ULx Clear Task.vi"("task in"=w238, "error in"=w240) -> ()  [unwired: 13 in, 1 out]
              }
            }
          }
          event "SweepVDAC": Value Change {
            n179 = event-data() -> ()  [unwired: 1 in, 6 out]
            n180 = case shown="True" "SweepVDAC" {
              frame False {
              }
              frame True {
                w305 = u16 1 items=["Voltage", "Current"] ("Source Mode  (0: Voltage)")
                w307 = dbl[] []
                w320 = u16 1 items=["Voltage", "Current"] ("Source Mode  (0: Voltage)")
                w324 = u16 1 items=["Volts", "Current", "Resistance"] ("Function (0: Volts)")
                w326 = u16 0 items=["Volts", "Current", "Resistance"] ("Function (0: Volts)")
                n181 = call <instrlib>:"Initialize.vi"("ID Query (True)"=FALSE, "VISA resource name"="Current source") -> ("error out"=w312:errorcluster, "VISA resource name out"=w313:refnum<visa-resource-name>)  [unwired: 8 in]
                n182 = call <instrlib>:"Configure Measurement.vi"("error in (no error)"=w312, "Enable Auto Range (T:Enable)"=TRUE, "Function (0: Volts)"=w326, "VISA resource name"=w313) -> ("error out"=w327:errorcluster, "VISA resource name out"=w328:refnum<visa-resource-name>)  [unwired: 6 in]
                n183 = call <instrlib>:"Configure Measurement.vi"("Manual Range (1.0)"=1e-07, "error in (no error)"=w327, "Enable Auto Range (T:Enable)"=FALSE, "Function (0: Volts)"=w324, "VISA resource name"=w328) -> ("error out"=w322:errorcluster, "VISA resource name out"=w321:refnum<visa-resource-name>)  [unwired: 5 in]
                n184 = call-poly <vilib>:"Ramp Pattern.vi"("start"="VDAC Min", "end"="VDAC Max", "delta"="VDAC Step") -> ("Ramp Pattern"=w309:dbl[])  [unwired: 6 in, 2 out]
                n185 = local read "Oversample"() -> (w306:i32)
                n186 = local read "Detector Resource"() -> (w308:refnum<visa-resource-name>)
                n187 = call <instrlib>:"Configure Output.vi"("Source Mode  (0: Voltage)"=w320, "error in (no error)"=w322, "Output Level (0)"="ISource", "VISA resource name"=w321) -> ("error out"=w319:errorcluster, "VISA resource name out"=w318:refnum<visa-resource-name>)  [unwired: 6 in]
                n188 = call <instrlib>:"Enable Output.vi"("error in (no error)"=w319, "Enable Output (T: Enable)"=TRUE, "VISA resource name"=w318) -> ("error out"=w315:errorcluster, "VISA resource name out"=w316:refnum<visa-resource-name>)  [unwired: 7 in]
                n189 = for {
                  tunnel: w316 -> [w332]
                  tunnel: w315 -> [w363]
                  tunnel: w309 -> [w362] mode=indexing
                  tunnel: [w332] -> w304
                  tunnel: [w354] -> w302
                  shift-right: [w357] -> _
                  shift-left: w307 -> [w359]
                  tunnel: w309 -> [w345]
                  tunnel: w308 -> [w331]
                  shift-right: [w347] -> _
                  shift-left: w307 -> [w349]
                  shift-right: [w346] -> _
                  shift-left: w307 -> [w348]
                  tunnel: w306 -> [w335]
                  tunnel: "Detector 5" -> [w333]
                  stop <- "Abort SweepVDAC" stop-if-true
                  w350 = u16 2 items=["High", "Med", "Low"] ("Gain")
                  w351 = u16 1 items=["High", "Med", "Low"] ("Gain")
                  w360 = u16 0 items=["High", "Med", "Low"] ("Gain")
                  n190 = call <instrlib>:"Set DAC.vi"("error in (no error)"=w363, "value (0)"=w362, "chan (0)"=w333, "VISA resource name"=w331) -> ("error out"=w361:errorcluster, "VISA resource name out"=w330:refnum<visa-resource-name>)  [unwired: 6 in]
                  n191 = call <instrlib>:"Get ADC.vi"("Gain"=w360, "Detector"=w333, "error in (no error)"=w361, "VISA resource name"=w330) -> ("error out"=w356:errorcluster, "output"=w358:i32, "VISA resource name out"=w353:refnum<visa-resource-name>)  [unwired: 5 in]
                  n192 = Divide(x=w358, y=w335) -> (x/y=w339:dbl)
                  n193 = call <instrlib>:"Get ADC.vi"("Gain"=w351, "Detector"=w333, "error in (no error)"=w356, "VISA resource name"=w353) -> ("error out"=w355:errorcluster, "output"=w338:i32, "VISA resource name out"=w352:refnum<visa-resource-name>)  [unwired: 5 in]
                  n194 = Divide(x=w338, y=w335) -> (x/y=w337:dbl)
                  n195 = call <instrlib>:"Get ADC.vi"("Gain"=w350, "Detector"=w333, "error in (no error)"=w355, "VISA resource name"=w352) -> ("error out"=w354:errorcluster, "output"=w334:i32)  [unwired: 5 in, 1 out]
                  n196 = Divide(x=w334, y=w335) -> (x/y=w336:dbl)
                  n197 = Build Array (concatenate)(w349, w337) -> (w347:dbl[])
                  n198 = Build Array (concatenate)(w359, w339) -> (w357:dbl[])
                  n199 = Build Array (concatenate)(w348, w336) -> (w346:dbl[])
                  n200 = Bundle("Ramp Pattern"=w345, w357) -> (w344:cluster{"Ramp Pattern":dbl[], dbl[]})  [unwired: 1 in]
                  n201 = Bundle("Ramp Pattern"=w345, w347) -> (w343:cluster{"Ramp Pattern":dbl[], dbl[]})  [unwired: 1 in]
                  n202 = Bundle("Ramp Pattern"=w345, w346) -> (w342:cluster{"Ramp Pattern":dbl[], dbl[]})  [unwired: 1 in]
                  n203 = Build Array(w344, w343, w342) -> (→"VDAC Sweep":cluster{"Ramp Pattern":dbl[], dbl[]}[])
                }
                n204 = call <instrlib>:"Configure Output.vi"("Source Mode  (0: Voltage)"=w305, "error in (no error)"=w302, "Output Level (0)"=0.0, "VISA resource name"=w304) -> ("error out"=w301:errorcluster, "VISA resource name out"=w303:refnum<visa-resource-name>)  [unwired: 6 in]
                n205 = call <instrlib>:"Enable Output.vi"("error in (no error)"=w301, "Enable Output (T: Enable)"=FALSE, "VISA resource name"=w303) -> ("error out"=w311:errorcluster, "VISA resource name out"=w310:refnum<visa-resource-name>)  [unwired: 7 in]
                n206 = call <instrlib>:"Close.vi"("error in (no error)"=w311, "VISA resource name"=w310) -> ()  [unwired: 9 in, 1 out]
              }
            }
          }
          event "Step": Value Change {
            n207 = event-data() -> ()  [unwired: 1 in, 6 out]
            n208 = case shown="True" "Step" {
              frame False {
              }
              frame True {
                w376 = 1000 ("oversample (0)")
                w388 = u16 1 items=["Voltage", "Current"] ("Source Mode  (0: Voltage)")
                w392 = u16 1 items=["Voltage", "Current"] ("Source Mode  (0: Voltage)")
                w395 = u16 1 items=["Volts", "Current", "Resistance"] ("Function (0: Volts)")
                w398 = u16 0 items=["Volts", "Current", "Resistance"] ("Function (0: Volts)")
                n209 = local read "Detector Resource"() -> (w372:refnum<visa-resource-name>)
                n210 = property on="Oversample" class="DigNum (strict)"() -> (error out=w384:errorcluster, "Value"=w367:i32)  [unwired: 2 in, 1 out]
                n211 = call <instrlib>:"Set OverSample.vi"("error in (no error)"=w384, "oversample (0)"=w376, "VISA resource name"=w372) -> ("error out"=w385:errorcluster)  [unwired: 7 in, 1 out]
                n212 = local read "Current source"() -> (w365:refnum<visa-resource-name>)
                n213 = call <instrlib>:"Initialize.vi"("error in (no error)"=w385, "ID Query (True)"=FALSE, "VISA resource name"=w365) -> ("error out"=w408:errorcluster, "VISA resource name out"=w407:refnum<visa-resource-name>)  [unwired: 7 in]
                n214 = call <instrlib>:"Configure Measurement.vi"("error in (no error)"=w408, "Enable Auto Range (T:Enable)"=TRUE, "Function (0: Volts)"=w398, "VISA resource name"=w407) -> ("error out"=w402:errorcluster, "VISA resource name out"=w401:refnum<visa-resource-name>)  [unwired: 6 in]
                n215 = call <instrlib>:"Configure Measurement.vi"("Manual Range (1.0)"=1e-07, "error in (no error)"=w402, "Enable Auto Range (T:Enable)"=FALSE, "Function (0: Volts)"=w395, "VISA resource name"=w401) -> ("error out"=w403:errorcluster, "VISA resource name out"=w404:refnum<visa-resource-name>)  [unwired: 5 in]
                n216 = call <instrlib>:"Configure Output.vi"("Source Mode  (0: Voltage)"=w392, "error in (no error)"=w403, "Output Level (0)"="Current 1", "VISA resource name"=w404) -> ("error out"=w405:errorcluster, "VISA resource name out"=w406:refnum<visa-resource-name>)  [unwired: 6 in]
                n217 = call <instrlib>:"Enable Output.vi"("error in (no error)"=w405, "Enable Output (T: Enable)"=TRUE, "VISA resource name"=w406) -> ("error out"=w391:errorcluster, "VISA resource name out"=w387:refnum<visa-resource-name>)  [unwired: 7 in]
                n218 = call <userlib>:"Wait (ms)__ogtk.vi"("error in (no error)"=w391, "milliseconds to wait"="Delay 1 (ms)") -> ("error out"=w389:errorcluster)  [unwired: 8 in, 1 out]
                n219 = call <instrlib>:"Configure Output.vi"("Source Mode  (0: Voltage)"=w388, "error in (no error)"=w389, "Output Level (0)"="Current 2", "VISA resource name"=w387) -> ("error out"=w383:errorcluster, "VISA resource name out"=w369:refnum<visa-resource-name>)  [unwired: 6 in]
                n220 = call <instrlib>:"Get BURST.vi"("error in (no error)"=w383, "chan (0)"="chan (0)", "VISA resource name"=w372) -> ("error out"=w381:errorcluster, "subarray"=w374:dbl[], "VISA resource name out"=w380:refnum<visa-resource-name>)  [unwired: 5 in, 1 out]
                n221 = for {
                  tunnel: w374 -> [_] mode=indexing
                  tunnel: [w409] -> w379 mode=indexing
                  i -> [w409]
                }
                n222 = call <instrlib>:"Get Time.vi"("error in (no error)"=w381, "VISA resource name"=w380) -> ("error out"=w370:errorcluster, "output"=w378:i32, "VISA resource name out"=w366:refnum<visa-resource-name>)  [unwired: 7 in]
                n223 = Divide(x=w378, y=w376) -> (x/y=w377:dbl)
                n224 = Multiply(x=w377, y=w379) -> (x*y=w375:dbl[])
                n225 = Bundle(w375, "subarray"=w374) -> (→"Step Response":cluster{dbl[], "subarray":dbl[]})  [unwired: 1 in]
                n226 = call <instrlib>:"Enable Output.vi"("error in (no error)"=w370, "Enable Output (T: Enable)"=TRUE, "VISA resource name"=w369) -> ("error out"=w368:errorcluster)  [unwired: 7 in, 1 out]
                n227 = call <instrlib>:"Set OverSample.vi"("error in (no error)"=w368, "oversample (0)"=w367, "VISA resource name"=w366) -> ()  [unwired: 7 in, 2 out]
              }
            }
          }
          event "Exit": Value Change {
            # "If stage is connected, go to reference position and then exit"
            n228 = event-data() -> ()  [unwired: 1 in, 6 out]
          }
          event Panel Close? {
            # "Discard \"Panel Close?\" event\n\nto leave program through\n graceful route"
            # "NOTE:\nMake sure not to use the red \"Abort Execution\" button in the\nLabVIEW menu to abort the application execution.\nDoing so will not close the device connection with the consequence that\na re-open after the next application start will fail."
            # "\"Panel Close\" (\"X\") was clicked by the user:\nWe discard the close command and set an \"exit\" flag. This gives us the change to proper disconnect the device and clean up the application before closing the window."
            # "Trap \"Panel Close\" instruction and exit program gracefully"
            n229 = event-data() -> ()  [unwired: 1 in, 4 out]
            n230 = local write "exit"(TRUE ("exit")) -> ()
            n231 = event-data("Discard?"=TRUE) -> ()  [unwired: 1 in, 1 out]
          }
        }
      }
    }
    frame #2 {
      # "Also power off and close detector SCPI EGSE"
      # "Cleanup and Shutdown"
      n232 = local read "Detector Resource"() -> (w417:refnum<visa-resource-name>)
      n233 = call <instrlib>:"Set Power.vi"("Power (0)"=FALSE, "VISA resource name"=w417) -> ("error out"=w414:errorcluster, "VISA resource name out"=w418:refnum<visa-resource-name>)  [unwired: 8 in]
      n234 = property on="Power" class="Bool (strict)"(error in=w414, "Value"=FALSE ("Power")) -> (error out=w415:errorcluster)  [unwired: 1 in, 1 out]
      n235 = call <instrlib>:"Close.vi"("error in (no error)"=w415, "VISA resource name"=w418) -> ()  [unwired: 9 in, 1 out]
    }
  }
  "error out" <- w1
